vi "DAQvero.vi"(0 "task/channels in":refnum<k21>, 1 "sampling info":cluster{"Fs":dbl, "#s":dbl}={"Fs"=10000.0, "#s"=1000.0}, 2 "error in":errorcluster) -> (3 "task out":refnum<k21>, 4 "1 segnale":waveform(dbl)={"t0"=timestamp(42.1 s since 1904-01-01), "dt"=0.0001, "Y"=array[1000 elements]}, 5 "2 segnale":waveform(dbl)={"t0"=timestamp(42.1 s since 1904-01-01), "dt"=0.0001, "Y"=array[1000 elements]}, 6 "error out":errorcluster)   [LabVIEW 2018]
uses:
  <vilib>/DAQmx/read.llb/DAQmx Read (Analog 1D Wfm NChan NSamp).vi
  <vilib>/DAQmx/configure/timing.llb/DAQmx Timing (Sample Clock).vi
  <vilib>/DAQmx/miscellaneous.llb/DAQmx Fill In Error Info.vi
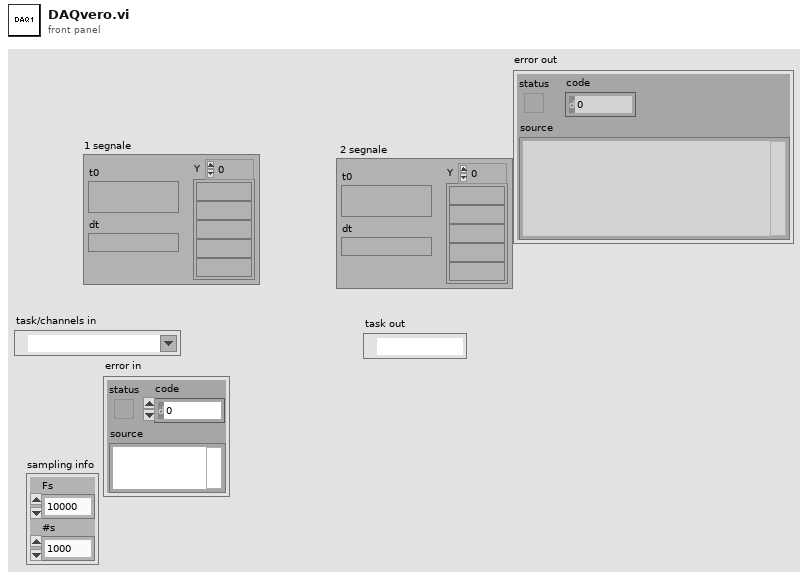
[diagram p1: front panel]
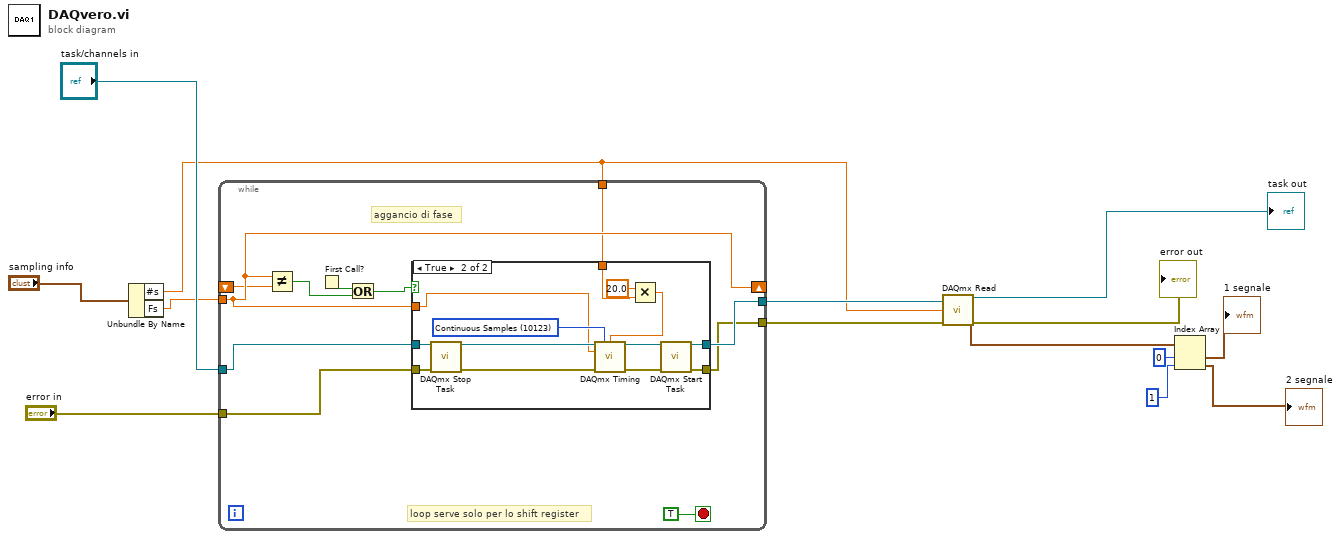
[diagram p0: block diagram]
diagram:
  n1 = Unbundle By Name("sampling info") -> ("#s"=w1:dbl, "Fs"=w2:dbl)
  n2 = while {
    shift-right: [w17] -> _
    shift-left: _ -> [w16]
    tunnel: w2 -> [w17]
    tunnel: "error in" -> [w25]
    tunnel: "task/channels in" -> [w24]
    tunnel: [w22] -> w4
    tunnel: [w21] -> w3
    tunnel: w1 -> [w15]
    stop <- TRUE stop-if-true
    # "aggancio di fase"
    # "loop serve solo per lo shift register"
    n3 = Not Equal?(x=w17, y=w16) -> (x != y?=w20:bool)
    n4 = First Call?() -> (First Call?: T/F=w23:bool)
    n5 = Or(x=w23, y=w20) -> (x .or. y?=w19:bool)
    n6 = case shown="True" w19 {
      tunnel: w17 -> [_ w31]
      tunnel: w25 -> [w26 w36]
      tunnel: w24 -> [w27 w37]
      tunnel: [w27 w35] -> w22
      tunnel: [w26 w34] -> w21
      tunnel: w15 -> [_ w30]
      frame False {
      }
      frame True {
        w40 = 10123 items=["Finite Samples"=10178, "Continuous Samples"=10123, "Hardware Timed Single Point"=12522] ("sample mode")
        n7 = call <vilib>:"DAQmx Stop Task.vi"("task/channels in"=w37, "error in"=w36) -> ("task out"=w39:refnum<k21>, "error out"=w38:errorcluster)  [unwired: 12 in]
        n8 = Multiply(x=20.0 ("y"), y=w30) -> (x*y=w28:dbl)
        n9 = call-poly <vilib>:"DAQmx Timing.vi"("task/channels in"=w39, "sample mode"=w40, "samples per channel"=w28, "rate"=w31, "error in"=w38) -> ("task out"=w33:refnum<k21>, "error out"=w32:errorcluster)  [unwired: 9 in]
        n10 = call <vilib>:"DAQmx Start Task.vi"("task/channels in"=w33, "error in"=w32) -> ("task out"=w35:refnum<k21>, "error out"=w34:errorcluster)  [unwired: 12 in]
      }
    }
  }
  n11 = call-poly <vilib>:"DAQmx Read.vi"("task/channels in"=w4, "number of samples per channel"=w1, "error in"=w3) -> ("task out"=→"task out":refnum<k21>, "data"=w13:waveform(dbl)[], "error out"=→"error out":errorcluster)  [unwired: 10 in]
  n12 = Index Array(array=w13, index #1=0 ("index"), index #2=1 ("index")) -> (element #1=→"1 segnale":waveform(dbl), element #2=→"2 segnale":waveform(dbl))
